vi "No Error.vi"() -> ()   [LabVIEW 2017, in "Assertion.Tests.lvlib" / "Assert Error Code.lvlib"]
uses:
  Assert Error Code.lvlib
  c1be48e0-8893-4c09-ba40-1e86d22c716c.vi
  Constraint/IsEqual/Create.vi
  Constraint/IsEqual/IsEqual.lvclass
  Assertion/Assertion.lvlib
panel:
  out "error out":errorcluster
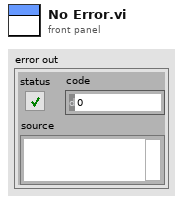
[diagram p1: front panel]
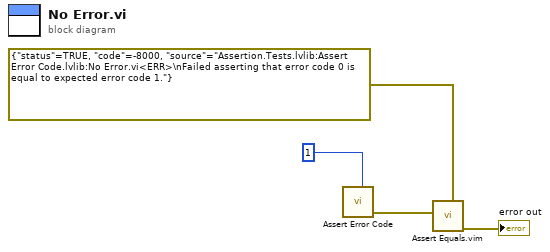
[diagram p0: block diagram]
diagram:
  n1 = call "Assert Error Code.vi"("Expected"=1) -> ("error out"=w3:errorcluster)  [unwired: 10 in]
  n2 = call "Assert Equals.vim"("Expected"=errorcluster {"status"=TRUE, "code"=-8000, "source"="Assertion.Tests.lvlib:Assert Error Code.lvlib:No Error.vi<ERR>\nFailed asserting that error code 0 is equal to expected error code 1."} ("error out 2"), "Actual"=w3) -> ("error out"=→"error out":errorcluster)  [unwired: 9 in]
